vi "Populate Registry.vi"(8 "error in":errorcluster, 10 "Aliases":string[](array[string]), 11 "Names":string[](array[string])) -> (0 "error out":errorcluster)   [LabVIEW 2019, in "Identifier.lvclass"]
uses:
  Identifier.lvclass
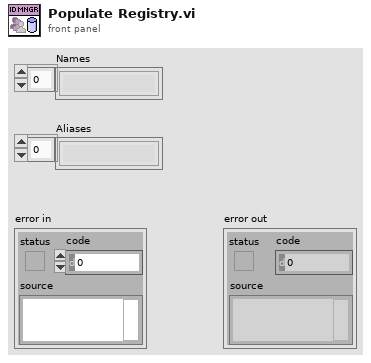
[diagram p1: front panel]
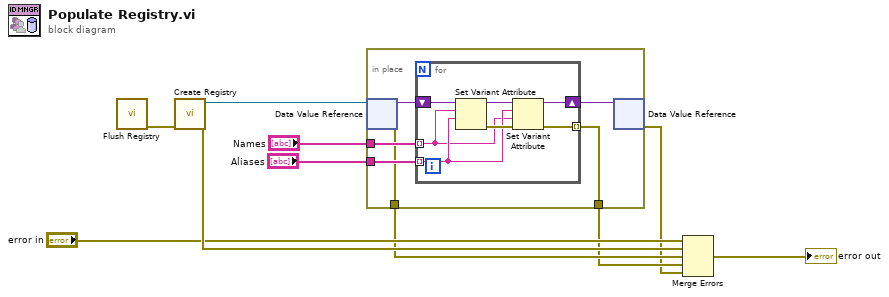
[diagram p0: block diagram]
diagram:
  n1 = call "Flush Registry.vi"() -> ("error out"=w6:errorcluster)  [unwired: 11 in]
  n2 = call "Create Registry.vi"("error in"=w6) -> ("error out"=w7:errorcluster, "Registry"=w10:refnum<data-value>)  [unwired: 9 in]
  n3 = in-place {
    in-place-border: "Names" -> [w14]
    in-place-border: "Aliases" -> [w13]
    in-place-border: [w12] -> w4
    in-place-border: [w11] -> w3
    n4 = in-place-dvr #1(w10) -> (w16:variant, w12:errorcluster)
    n5 = for {
      shift-right: [w21] -> w15
      shift-left: w16 -> [w23]
      tunnel: w14 -> [w18] mode=indexing
      tunnel: w13 -> [w19] mode=indexing
      tunnel: [w17] -> w11 mode=indexing
      n6 = Set Variant Attribute(Variant=w23, name=w18, value=w19) -> (Variant out=w22:variant, error out=w20:errorcluster)  [unwired: 1 in, 1 out]
      n7 = Set Variant Attribute(Variant=w22, name=w19, value=w18, error in=w20) -> (Variant out=w21:variant, error out=w17:errorcluster)  [unwired: 1 out]
    }
    n8 = in-place-dvr #1(w15) -> (w2:errorcluster)  [unwired: 1 out]
  }
  n9 = Merge Errors("error in", w7, w4, w3, w2) -> (→"error out":errorcluster)
